vi "Cache.Move.vi"(7 "Idx":i32, 8 "error in":errorcluster, 9 "Time (now)":timestamp, 10 "file":path, 11 "Data in":T1) -> (0 "error out":errorcluster, 3 "Data out":T1)   [LabVIEW 2016]
uses:
  Cache.Data.ctl
  Cache.Data.Status.ctl
  Cache.Data.Sets.ctl
  Tools/EventLog/EventLog.EventSource.ctl
  Tools/Translator/Translator.Message.ctl
  Tools/EventLog/EventLog.New(single).vi
  Global/ApplicationGlobal.vi
  Tools/EventLog/EventLog.Buffer.vi
  Tools/EventLog/EventLog.File.ReadWrite.vi
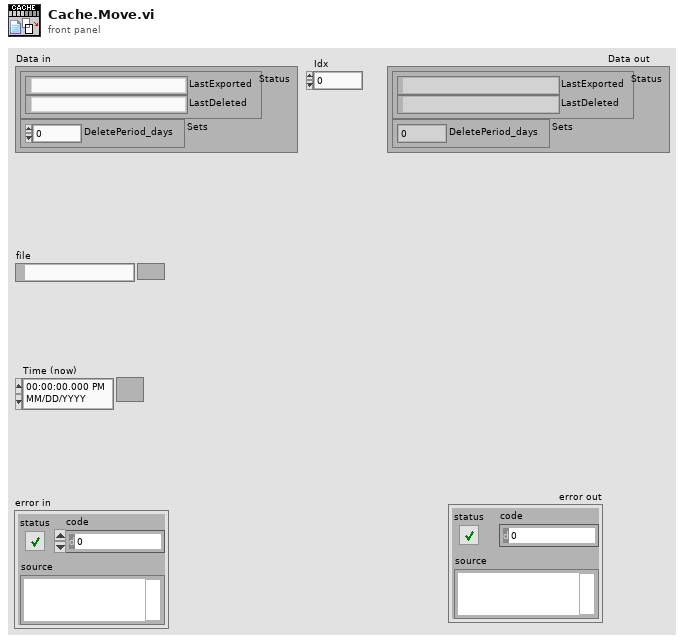
[diagram p1: front panel]
types:
  T1 = typedef "Cache.Data.ctl" = cluster{"Status":T2, "Sets":T3}
  T2 = typedef "Cache.Data.Status.ctl" = cluster{"LastExported":string, "LastDeleted":string}
  T3 = typedef "Cache.Data.Sets.ctl" = cluster{"DeletePeriod_days":dbl}
  T4 = typedef "Translator.Message.ctl" = enum16{"-", "Event confirmed", "Log out", "Log in", "Shutdown", "Cancel", "Start", "Continue", "Stop", "On", "Off", "OK", "NOK", "NOK %s", "This", "Prev", "Home", "Work", "In progress...", "Missing", "Empty", "Hardware failure", "Initial", "Error %d >> %s", "Error %d >> %s >> %s", "Starting %s", "Quitting %s", "Configured", "Initializing", "Quitting", "Loading", "Running %s", "Stopped", "Summary", "Do you want to continue?", "Do you want to exit?", "Log out?", "System", "All", "IDLE", "Translating...%s", "Not found", "Alarm %s", "Run", "Skip", "Abort", "Repeat", "Please wait...", "Database disconnected", "Login to database successful", "Login to database failed: %d; %s", "Get process step data for %s", "Changeover off", "Changeover into %s", "Product %s | %s found in cache with status %d at previous station", "Product %s | %s found in database with status %d at previous station", "Product %s | %s not found in cache at previous station", "Product %s | %s not found in database at previous station", "Product %s | %s found in cache with status %d at this station (%d repetion)", "Product %s | %s found in database with status %d at this station (%d repetition)", "Product %s | %s not found in cache at this station", "Product %s | %s not found in database at this station", "Product %s | %s found in cache for component %s | %s", "Product %s | %s found in database for component %s | %s", "Product not found in cache for component %s | %s", "Product not found in database for component %s | %s", "Product %s | %s connected with component %s | %s (cache)", "Product %s | %s connected with component %s | %s (database)", "New data for %s | %s (cache)", "New data for %s | %s (database)", "File %s moved (cache)", "File %s deleted (cache)", "Msg %d >> %s", "PLC LifeBit Failure", "Reconnecting DB", "Reconnecting PLC", "Free disk space is below 1GB - contact technician"}
  T5 = typedef "EventLog.EventSource.ctl" = enum16{"All", "Gui", "Cache", "PLC1", "PLC2", "PLC3", "DB", "DB01", "DB02", "DB03", "DB04", "DB05", "DB06", "DB07", "DB08", "DB09", "DB10", "DB11", "DB12", "DB13", "DB14", "DB15", "DB16"}
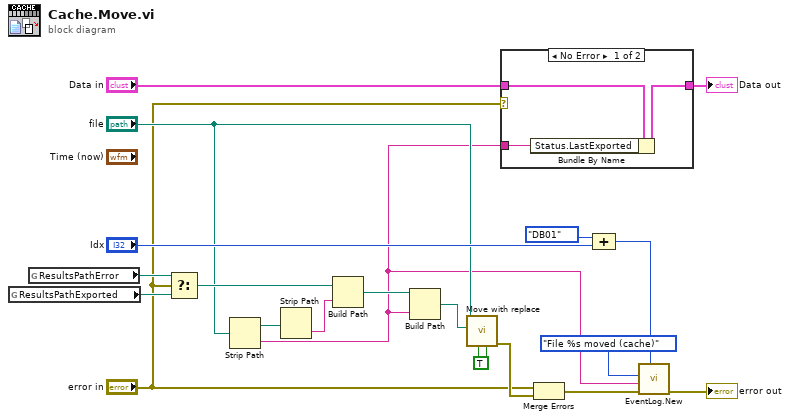
[diagram p0: block diagram]
diagram:
  w16 = TRUE ("create parent dirs (F)")
  n1 = global read "ApplicationGlobal.vi" "ResultsPathExported"() -> (w20:path)
  n2 = global read "ApplicationGlobal.vi" "ResultsPathError"() -> (w19:path)
  n3 = Select(t=w19, s="error in", f=w20) -> (s? t:f=w18:path)
  n4 = Strip Path(path="file") -> (stripped path=w8:path, name=w1:string)
  n5 = Strip Path(path=w8) -> (name=w6:string)  [unwired: 1 out]
  n6 = Build Path(base path=w18, name or relative path=w6) -> (appended path=w17:path)
  n7 = Build Path(base path=w17, name or relative path=w1) -> (appended path=w5:path)
  n8 = call "Move with replace.vi"("create parent dirs (F)"=w16, "replace allowed (T)"=w16, "destination path"=w5, "source path"="file") -> ("error"=w14:errorcluster)  [unwired: 7 in]
  n9 = case shown="No Error" "error in" {
    tunnel: "Data in" -> [w23 w24]
    tunnel: [w22 w24] -> w3
    tunnel: w1 -> [w21 _]
    frame No Error {
      n10 = Bundle By Name(cluster=w23, "Status.LastExported"=w21) -> (w22:T1)
    }
    frame Error {
    }
  }
  "Data out" <- w3
  n11 = Merge Errors("error in", w14) -> (w13:errorcluster)
  n12 = Compound Arithmetic op=ADD(EventLog.EventSource."DB01" ("Source (All)"), "Idx") -> (w9:i32)
  n13 = call-poly "EventLog.New.vi"("Source (All)"=w9, "error in (no error)"=w13, "Arg"=w1, "Message (-)"=Translator.Message."File %s moved (cache)") -> ("error out"=→"error out":errorcluster)  [unwired: 6 in, 1 out]
